vi "Ref_Temp_Calc.vi"(10 "Temp Array":dbl[](array[numeric])) -> (2 "T Ref":dbl)   [LabVIEW 2014]
panel:
  out "Total Time":i32
  out "Total Equiv Time":dbl
  # "Ref Temperature Calculation"
  # "Ref Temp calculated as per the EPA legislation\nUsing an R factor of 17500"
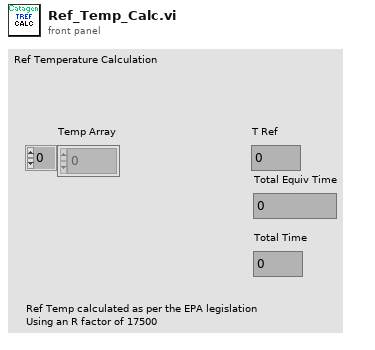
[diagram p1: front panel]
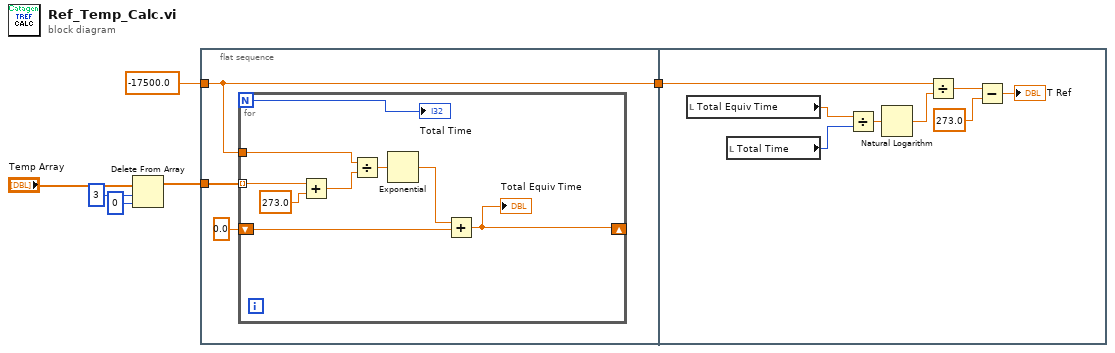
[diagram p0: block diagram]
diagram:
  n1 = Delete From Array(array="Temp Array", length=3, index=0) -> (array with subset deleted=w4:dbl[])  [unwired: 1 out]
  n2 = flat-sequence {
    tunnel: w4 -> [w9]
    tunnel: -17500.0 ("y") -> [w7]
    tunnel: [w7] -> w5
    tunnel: w5 -> [w26]
    frame #0 {
      n3 = for {
        N -> [w11]
        tunnel: w9 -> [w17] mode=indexing
        shift-right: [w13] -> _
        shift-left: 0.0 -> [w12]
        tunnel: w7 -> [w10]
        n4 = Add(x=w17, y=273.0) -> (x+y=w15:dbl)
        n5 = Divide(x=w10, y=w15) -> (x/y=w16:dbl)
        n6 = Exponential(1:w16) -> (0:w14:dbl)
        n7 = Add(x=w14, y=w12) -> (x+y=w13:dbl)
        "Total Equiv Time" <- w13
        "Total Time" <- w11
      }
    }
    frame #1 {
      n8 = local read "Total Equiv Time"() -> (w25:dbl)
      n9 = local read "Total Time"() -> (w24:i32)
      n10 = Divide(x=w25, y=w24) -> (x/y=w23:dbl)
      n11 = Natural Logarithm(1:w23) -> (0:w22:dbl)
      n12 = Divide(x=w26, y=w22) -> (x/y=w19:dbl)
      n13 = Subtract(x=w19, y=273.0) -> (x-y=→"T Ref":dbl)
    }
  }
